vi "SendCommands.vi"(8 "error in (no error)":errorcluster) -> (0 "error out":errorcluster)   [LabVIEW 2016]
uses:
  Global Variables/Master Ready For Data.vi
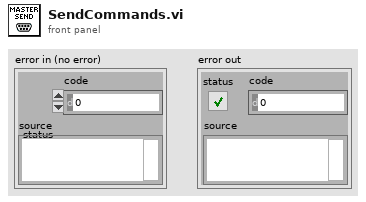
[diagram p1: front panel]
types:
  T1 = cluster{"Data":string, "Port":refnum<visa-resource-name>}
  T2 = cluster{"Data":string, "Port":refnum<visa-resource-name>}[]
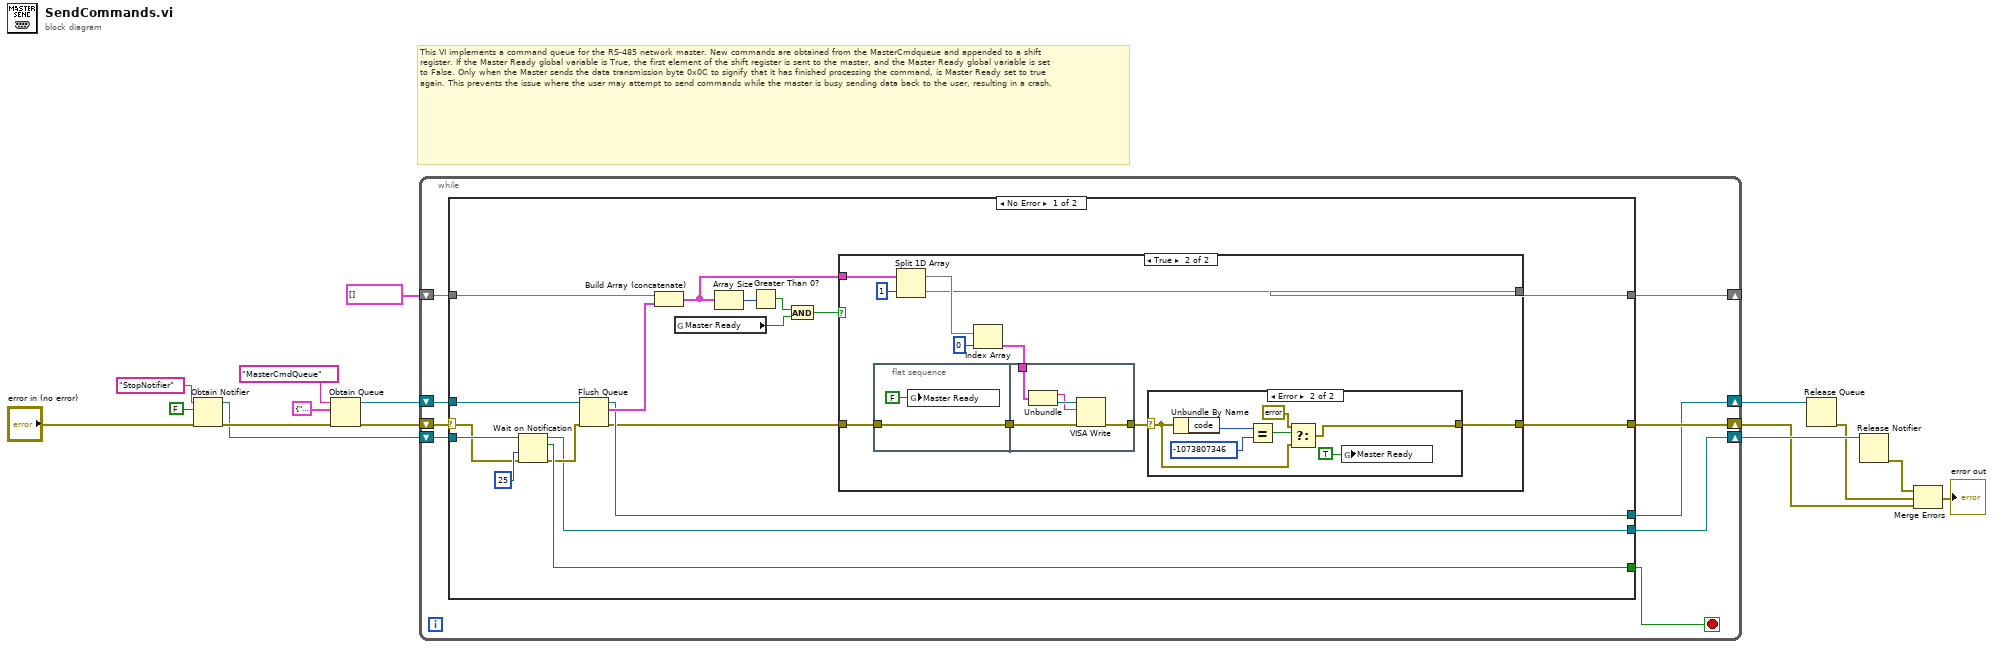
[diagram p0: block diagram]
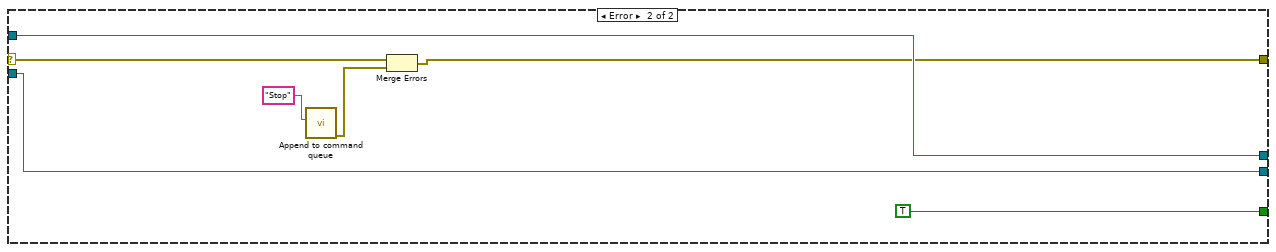
[diagram p4: hidden frame]
diagram:
  # "This VI implements a command queue for the RS-485 network master. New commands are obtained from the MasterCmdqueue and appended to a shift register. If the Master Ready global variable is True, the first element of the shift register is sent to the master, and the Master Ready global variable is set to False. Only when the Master sends the data transmission byte 0x0C to signify that it has finished processing the command, is Master Ready set to true again. This prevents the issue where the user may attempt to send commands while the master is busy sending data back to the user, resulting in a crash."
  n1 = Obtain Notifier(name (unnamed)="StopNotifier", notification data type=FALSE, error in (no error)="error in (no error)") -> (notifier out=w7:refnum<notifier>, error out=w9:errorcluster)  [unwired: 1 in, 1 out]
  n2 = Obtain Queue(name (unnamed)="MasterCmdQueue", element data type=T1 {"Data"="", "Port"=""} ("Cluster"), error in (no error)=w9) -> (queue out=w12:refnum<queue>, error out=w14:errorcluster)  [unwired: 2 in, 1 out]
  n3 = while {
    shift-right: [w21] -> _
    shift-left: T2 [] -> [w24]
    shift-right: [w17] -> w6
    shift-left: w7 -> [w22]
    shift-right: [w18] -> w5
    shift-left: w12 -> [w23]
    shift-right: [w25] -> w4
    shift-left: w14 -> [w20]
    stop <- w19 stop-if-true
    n4 = case shown="No Error" w20 {
      selector: w20 -> [w29 w72]
      tunnel: [w43 w71] -> w25
      tunnel: w24 -> [w38 _]
      tunnel: w23 -> [w37 w76]
      tunnel: w22 -> [w30 w75]
      tunnel: [w33 _] -> w21
      tunnel: [w32 TRUE] -> w19
      tunnel: [w31 w76] -> w18
      tunnel: [w27 w75] -> w17
      frame No Error {
        n5 = Wait on Notification(notifier=w30, timeout in ms (-1)=25, error in (no error)=w29) -> (notifier out=w27:refnum<notifier>, notification=w32:bool, error out=w28:errorcluster)  [unwired: 1 in, 1 out]
        n6 = Flush Queue(queue=w37, error in (no error)=w28) -> (queue out=w31:refnum<queue>, remaining elements=w36:T2, error out=w26:errorcluster)
        n7 = Build Array (concatenate)(w38, w36) -> (w35:T2)
        n8 = global read "Master Ready For Data.vi" "Master Ready"() -> (w40:bool)
        n9 = Array Size(array=w35) -> (size(s)=w42:i32)
        n10 = Greater Than 0?(x=w42) -> (x > 0?=w41:bool)
        n11 = And(x=w41, y=w40) -> (x .and. y?=w39:bool)
        n12 = case shown="True" w39 {
          tunnel: [w45 w46] -> w43
          tunnel: w26 -> [w45 w55]
          tunnel: w35 -> [w44 w53]
          tunnel: [w44 w50] -> w33
          frame False {
          }
          frame True {
            n13 = flat-sequence {
              tunnel: w55 -> [w65]
              tunnel: [w65] -> w54
              tunnel: [w70] -> w47
              tunnel: w54 -> [w69]
              tunnel: w48 -> [w66]
              frame #0 {
                n14 = global write "Master Ready For Data.vi" "Master Ready"(FALSE ("Master Ready")) -> ()
              }
              frame #1 {
                n15 = Unbundle(w66) -> ("Data"=w67:string, "Port"=w68:refnum<visa-resource-name>)
                n16 = VISA Write(VISA resource name=w68, write buffer=w67, error in (no error)=w69) -> (error out=w70:errorcluster)  [unwired: 2 out]
              }
            }
            n17 = Split 1D Array(array=w53, index=1) -> (first subarray=w51:T2, second subarray=w50:T2)
            n18 = Index Array(array=w51, index=0) -> (element=w48:T1)
            n19 = case shown="Error" w47 {
              selector: w47 -> [w56 w60]
              tunnel: [w56 w58] -> w46
              frame No Error {
              }
              frame Error {
                n20 = Unbundle By Name(w60) -> ("code"=w63:i32)
                n21 = Equal?(x=w63, y=-1073807346) -> (x = y?=w61:bool)
                n22 = Select(t=errorcluster {"status"=FALSE, "code"=0, "source"=""}, s=w61, f=w60) -> (s? t:f=w58:errorcluster)
                n23 = global write "Master Ready For Data.vi" "Master Ready"(TRUE ("Master Ready")) -> ()
              }
            }
          }
        }
      }
      frame Error {
        n24 = call "Append to command queue.vi"("Single command"="Stop") -> ("error out"=w73:errorcluster)  [unwired: 10 in]
        n25 = Merge Errors(w72, w73) -> (w71:errorcluster)
      }
    }
  }
  n26 = Release Queue(queue=w5) -> (error out=w3:errorcluster)  [unwired: 2 in, 2 out]
  n27 = Release Notifier(notifier=w6) -> (error out=w2:errorcluster)  [unwired: 2 in, 2 out]
  n28 = Merge Errors(w2, w3, w4) -> (→"error out":errorcluster)
